vi "PurePursuit.vi"(0 "PathData":T2={"Path"=[{"x"=20.453371592539455, "y"=249.15925394548063}, {"x"=32.451138071473615, "y"=249.2417431099791}, {"x"=44.448056211953954, "y"=249.32366698389004}, {"x"=56.441768980000354, "y"=249.4040828136747}, {"x"=68.42823711154045, "y"=249.48106130123531}, {"x"=80.3987950137465, "y"=249.55036007485356}, {"x"=92.33398719870449, "y"=249.6026243647297}, {"x"=104.19073617112089, "y"=249.61714678939316}, {"x"=115.8737280283298, "y"=249.54805321076083}, {"x"=127.17183717836993, "y"=249.29372430937337}, {"x"=137.61733743281803, "y"=248.62905317811618}, {"x"=146.1740836060984, "y"=247.05537254809167}, {"x"=150.54675993154666, "y"=243.46800813008085}, {"x"=152.39728417160754, "y"=235.46668065740275}, {"x"=152.95934006523578, "y"=225.71717171741398}, {"x"=152.6076327980232, "y"=215.7198087862704}, {"x"=151.107691158904, "y"=206.8096834259849}, {"x"=147.4595538788043, "y"=201.04671193240875}, {"x"=139.23112896790275, "y"=198.5372634006921}, {"x"=128.93601727531555, "y"=197.49649482245655}, {"x"=117.71002861894719, "y"=197.11868334076806}, {"x"=106.06838831868264, "y"=197.04007755842468}, {"x"=94.24922045605804, "y"=197.09639645188625}, {"x"=82.37229762541514, "y"=197.21330877376334}, {"x"=70.51888885096747, "y"=197.35687893558043}, {"x"=58.78593931213765, "y"=197.51094316379152}, {"x"=47.350700340581184, "y"=197.66633376164685}, {"x"=36.58889694113597, "y"=197.8147673041893}, {"x"=27.32521119491603, "y"=197.9433223158581}, {"x"=21.38307030129124, "y"=198.025824964132}], "Spacing"=12.0}, 1 "SensorData":T3={"LeftDistance"=0.0, "RightDistance"=0.0, "LeftVelocity"=78.75762159095939, "RightVelocity"=-76.3848555077329, "Angle"=-0.01, "Location"={11.691968699047118, 248.03471515703785}}, 3 "Trackwidth":dbl=40.0 format="%#_13g", 5 "LookAhead":dbl=15.0, 7 "Reset":bool, 9 "MaxVel":dbl=40.0, 12 "Max Accel":dbl=50.0 format="%#_13g", 14 "Gains":T4={"FFV"=0.0088, "FFA"=0.0017, "Vel PID"={"P"=0.02, "I"=0.0, "D"=0.0}} {"Vel PID"."D" format="%.3f"; "Vel PID"."I" format="%.3f"; "Vel PID"."P" format="%.3f"}) -> (2 "Graph":cluster{cluster{"x":dbl, "y":dbl}[]}[](graph)=[{[{"x"=20.453371592539455, "y"=249.15925394548063}, {"x"=32.451138071473615, "y"=249.2417431099791}, {"x"=44.448056211953954, "y"=249.32366698389004}, {"x"=56.441768980000354, "y"=249.4040828136747}, {"x"=68.42823711154045, "y"=249.48106130123531}, {"x"=80.3987950137465, "y"=249.55036007485356}, {"x"=92.33398719870449, "y"=249.6026243647297}, {"x"=104.19073617112089, "y"=249.61714678939316}, {"x"=115.8737280283298, "y"=249.54805321076083}, {"x"=127.17183717836993, "y"=249.29372430937337}, {"x"=137.61733743281803, "y"=248.62905317811618}, {"x"=146.1740836060984, "y"=247.05537254809167}, {"x"=150.54675993154666, "y"=243.46800813008085}, {"x"=152.39728417160754, "y"=235.46668065740275}, {"x"=152.95934006523578, "y"=225.71717171741398}, {"x"=152.6076327980232, "y"=215.7198087862704}, {"x"=151.107691158904, "y"=206.8096834259849}, {"x"=147.4595538788043, "y"=201.04671193240875}, {"x"=139.23112896790275, "y"=198.5372634006921}, {"x"=128.93601727531555, "y"=197.49649482245655}, {"x"=117.71002861894719, "y"=197.11868334076806}, {"x"=106.06838831868264, "y"=197.04007755842468}, {"x"=94.24922045605804, "y"=197.09639645188625}, {"x"=82.37229762541514, "y"=197.21330877376334}, {"x"=70.51888885096747, "y"=197.35687893558043}, {"x"=58.78593931213765, "y"=197.51094316379152}, {"x"=47.350700340581184, "y"=197.66633376164685}, {"x"=36.58889694113597, "y"=197.8147673041893}, {"x"=27.32521119491603, "y"=197.9433223158581}, {"x"=21.38307030129124, "y"=198.025824964132}]}, {[{"x"=11.691968699047118, "y"=248.03471515703785}, {"x"=23.691968516276667, "y"=248.03680955212963}]}, {[{"x"=152.95934006523578, "y"=225.71717171741398}]}, {[{"x"=26.691968699047116, "y"=248.03471515703785}, {"x"=25.95781644347442, "y"=252.66997007266207}, {"x"=23.827223614671333, "y"=256.85149394142496}, {"x"=20.508747483434213, "y"=260.16997007266207}, {"x"=16.32722361467133, "y"=262.3005629014651}, {"x"=11.69196869904712, "y"=263.03471515703785}, {"x"=7.056713783422908, "y"=262.3005629014651}, {"x"=2.875189914660023, "y"=260.16997007266207}, {"x"=-0.4432862165770928, "y"=256.85149394142496}, {"x"=-2.5738790453801847, "y"=252.66997007266207}, {"x"=-3.308031300952882, "y"=248.03471515703785}, {"x"=-2.5738790453801865, "y"=243.39946024141364}, {"x"=-0.44328621657709455, "y"=239.21793637265077}, {"x"=2.8751899146600195, "y"=235.89946024141364}, {"x"=7.056713783422905, "y"=233.76886741261055}, {"x"=11.691968699047115, "y"=233.03471515703785}, {"x"=16.327223614671325, "y"=233.76886741261055}, {"x"=20.508747483434213, "y"=235.89946024141364}, {"x"=23.82722361467133, "y"=239.21793637265074}, {"x"=25.95781644347442, "y"=243.39946024141364}, {"x"=26.691968699047116, "y"=248.03471515703785}]}, {[{"x"=16.728162111415877, "y"=242.99940064954055}, {"x"=16.48171627411582, "y"=244.55539842807914}, {"x"=15.766502597859695, "y"=245.95908430278035}, {"x"=14.652531180466154, "y"=247.0730557201739}, {"x"=13.248845305764926, "y"=247.78826939643002}, {"x"=11.692847527226334, "y"=248.03471523373008}, {"x"=10.136849748687744, "y"=247.78826939643002}, {"x"=8.733163873986515, "y"=247.0730557201739}, {"x"=7.619192456592972, "y"=245.95908430278035}, {"x"=6.903978780336848, "y"=244.55539842807914}, {"x"=6.6575329430367916, "y"=242.99940064954055}, {"x"=6.903978780336848, "y"=241.44340287100195}, {"x"=7.619192456592971, "y"=240.03971699630074}, {"x"=8.733163873986513, "y"=238.9257455789072}, {"x"=10.136849748687743, "y"=238.21053190265107}, {"x"=11.692847527226332, "y"=237.964086065351}, {"x"=13.248845305764924, "y"=238.21053190265107}, {"x"=14.652531180466152, "y"=238.9257455789072}, {"x"=15.766502597859695, "y"=240.03971699630074}, {"x"=16.48171627411582, "y"=241.44340287100195}, {"x"=16.728162111415877, "y"=242.99940064954055}]}], 4 "LeftValue":dbl=2.7501251582780792, 6 "RightValue":dbl=-2.0461251582780795, 8 "TargetVel":dbl=40.0, 10 "Done":bool)   [LabVIEW 2017]
doc: "Takes in encoder and gyro data, and a path. In real time, calculates the left and right power to send to the motors to travel the path at a specified max speed, acceleration, and lookahead distance"
panel:
  in  "Speed/Curve":dbl=3.0 format="%#_13g"
  in  "Max dx/dt":dbl=10.0 format="%#_13g"
  out "TargetVelGraph":dbl(graph)
  out "Waveform Chart":T1(graph)={"l"=198.87785889523798, "dx/dt"=78.75762159095939, "r"=-118.87785889523798, "dx/dt"=-76.3848555077329}
  in  "Average Vels":bool
  # "SET DEFAULTS"
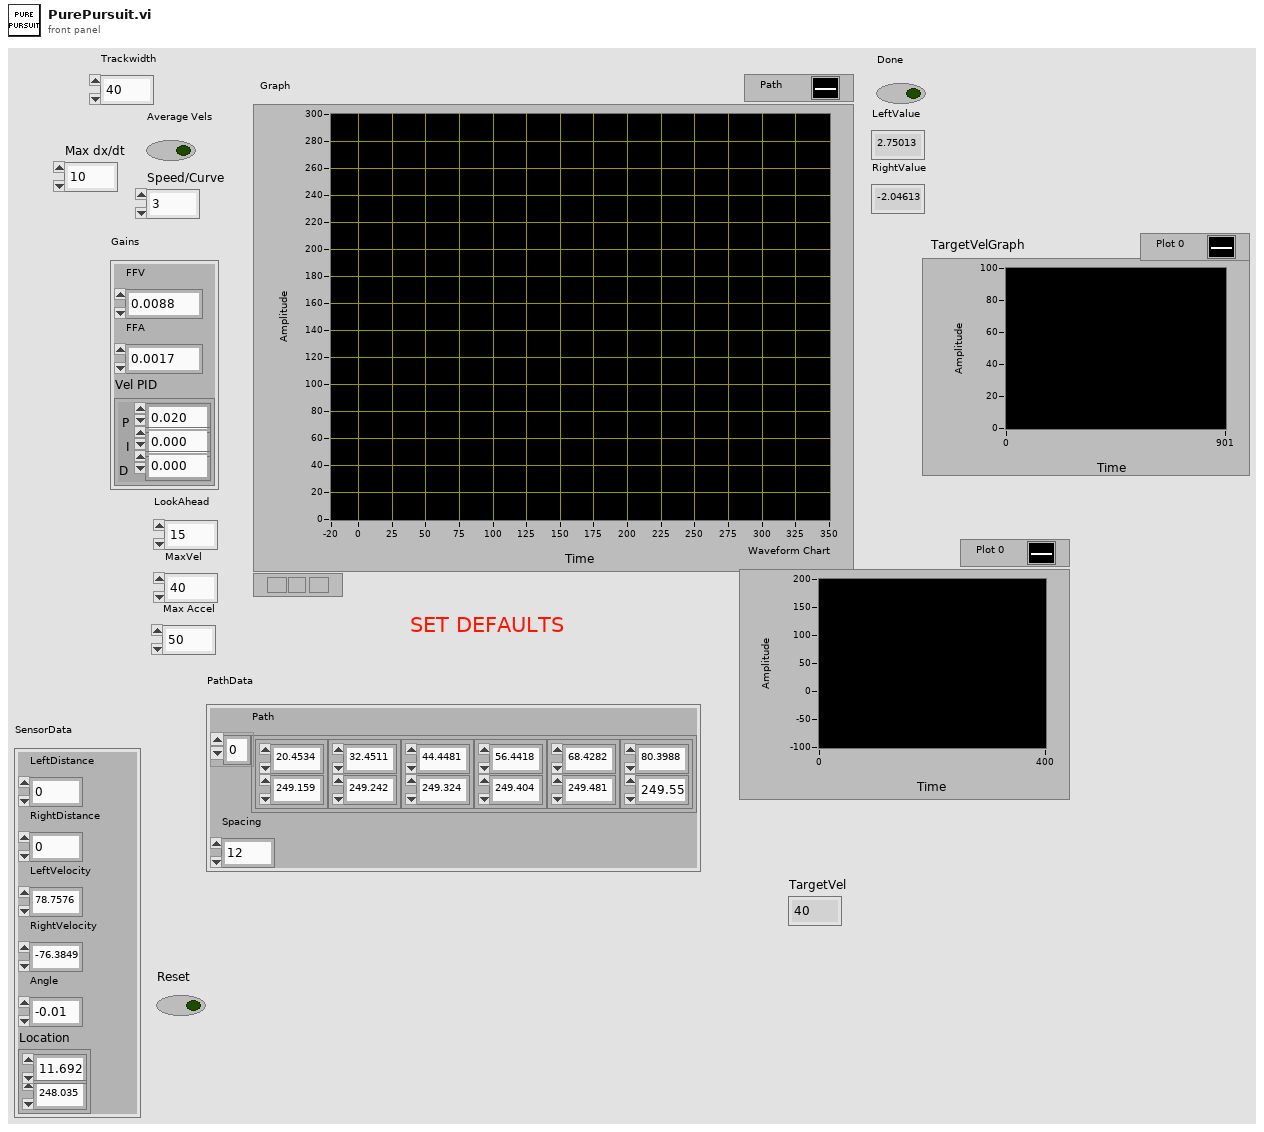
[diagram p1: front panel]
types:
  T1 = cluster{"l":dbl, "dx/dt":dbl, "r":dbl, "dx/dt":dbl}
  T2 = cluster{"Path":cluster{"x":dbl, "y":dbl}[], "Spacing":dbl}
  T3 = cluster{"LeftDistance":dbl, "RightDistance":dbl, "LeftVelocity":dbl, "RightVelocity":dbl, "Angle":dbl, "Location":cluster{dbl, dbl}}
  T4 = cluster{"FFV":dbl, "FFA":dbl, "Vel PID":cluster{"P":dbl, "I":dbl, "D":dbl}}
  T5 = cluster{"Path":cluster{"x":dbl, "y":dbl}[], "Spacing":dbl, "DistancesToEnd":dbl[], "Vel":dbl[]}
  T6 = cluster{"l":dbl, "LeftVelocity":dbl, "r":dbl, "RightVelocity":dbl}
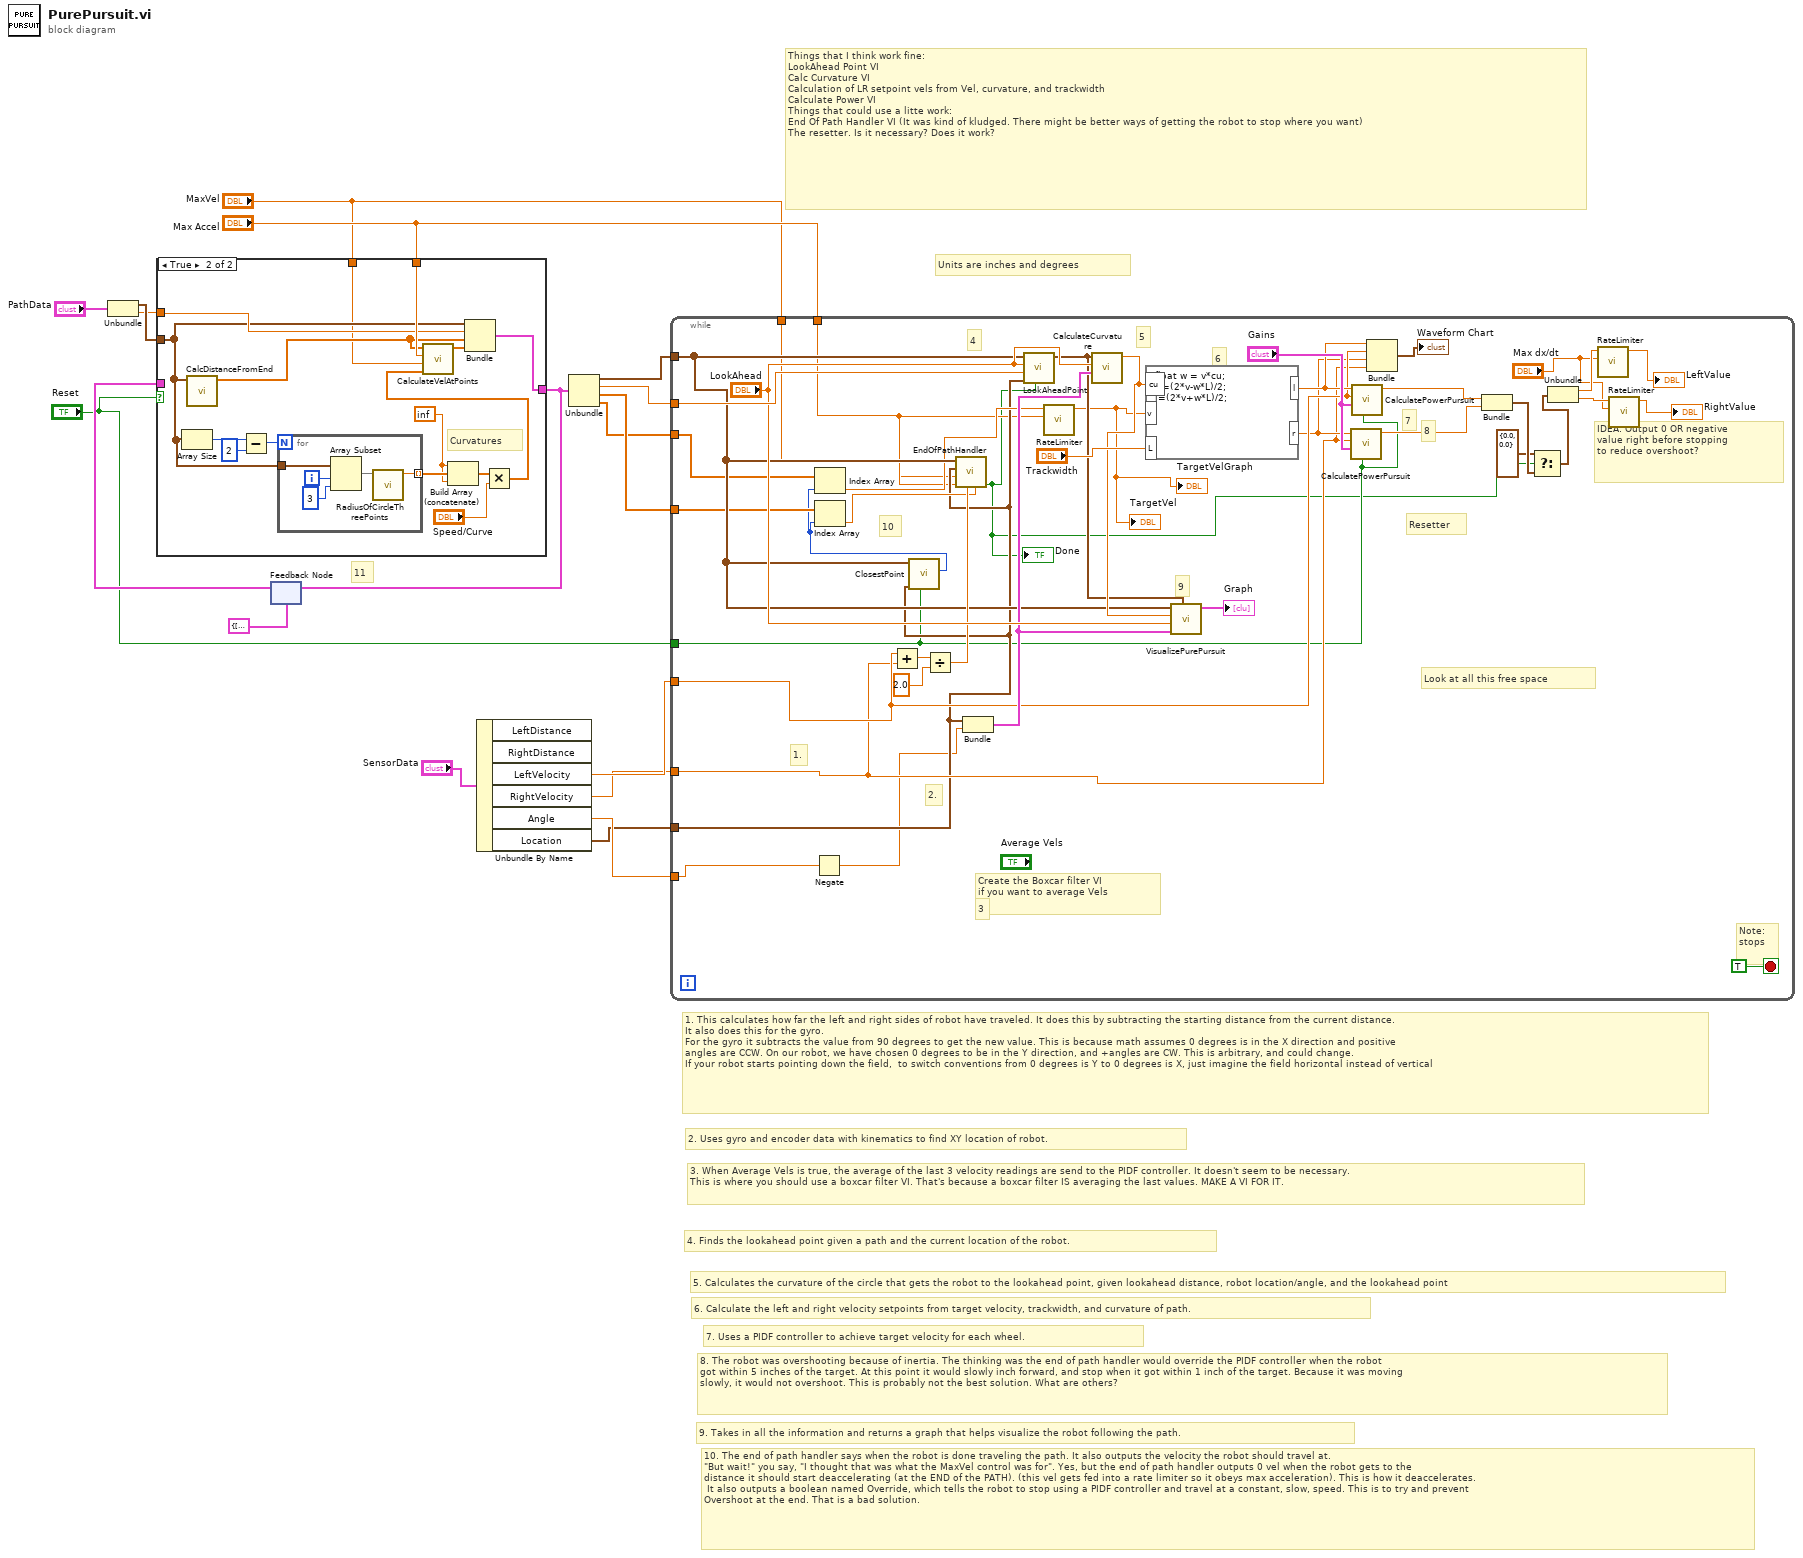
[diagram p0: block diagram]
diagram:
  # "11"
  # "10. The end of path handler says when the robot is done traveling the path. It also outputs the velocity the robot should travel at.\n\"But wait!\" you say, \"I thought that was what the MaxVel control was for\". Yes, but the end of path handler outputs 0 vel when the robot gets to the\ndistance it should start deaccelerating (at the END of the PATH). (this vel gets fed into a rate limiter so it obeys max acceleration). This is how it deaccelerates. \n It also outputs a boolean named Override, which tells the robot to stop using a PIDF controller and travel at a constant, slow, speed. This is to try and prevent\nOvershoot at the end. That is a bad solution."
  # "9. Takes in all the information and returns a graph that helps visualize the robot following the path."
  # "8. The robot was overshooting because of inertia. The thinking was the end of path handler would override the PIDF controller when the robot\ngot within 5 inches of the target. At this point it would slowly inch forward, and stop when it got within 1 inch of the target. Because it was moving\nslowly, it would not overshoot. This is probably not the best solution. What are others?"
  # "7. Uses a PIDF controller to achieve target velocity for each wheel."
  # "6. Calculate the left and right velocity setpoints from target velocity, trackwidth, and curvature of path."
  # "Things that I think work fine:\nLookAhead Point VI\nCalc Curvature VI\nCalculation of LR setpoint vels from Vel, curvature, and trackwidth\nCalculate Power VI\nThings that could use a litte work:\nEnd Of Path Handler VI (It was kind of kludged. There might be better ways of getting the robot to stop where you want)\nThe resetter. Is it necessary? Does it work?"
  # "Units are inches and degrees"
  # "5. Calculates the curvature of the circle that gets the robot to the lookahead point, given lookahead distance, robot location/angle, and the lookahead point"
  # "4. Finds the lookahead point given a path and the current location of the robot."
  # "3. When Average Vels is true, the average of the last 3 velocity readings are send to the PIDF controller. It doesn't seem to be necessary.\nThis is where you should use a boxcar filter VI. That's because a boxcar filter IS averaging the last values. MAKE A VI FOR IT."
  # "2. Uses gyro and encoder data with kinematics to find XY location of robot."
  # "1. This calculates how far the left and right sides of robot have traveled. It does this by subtracting the starting distance from the current distance.\nIt also does this for the gyro.\nFor the gyro it subtracts the value from 90 degrees to get the new value. This is because math assumes 0 degrees is in the X direction and positive\nangles are CCW. On our robot, we have chosen 0 degrees to be in the Y direction, and +angles are CW. This is arbitrary, and could change.\nIf your robot starts pointing down the field,  to switch conventions from 0 degrees is Y to 0 degrees is X, just imagine the field horizontal instead of vertical"
  n1 = Unbundle("PathData") -> ("Path"=w3:cluster{"x":dbl, "y":dbl}[], "Spacing"=w2:dbl)
  n2 = feedback #1(T5 {"Path"=[{"x"=0.0, "y"=0.0}, {"x"=0.0, "y"=46.0}, {"x"=77.25, "y"=97.5}], "Spacing"=0.0, "DistancesToEnd"=[309.52253206522465, 306.5225388483889, 303.52254576348514, 300.5225494135135, 297.5225482930251, 294.5225431892043, 291.52253649479525, 288.5225309404311, 285.52252839669825, 282.52252922985826, 279.52253236801363, 276.5225359199274, 273.5225380077533, 270.5225374640896, 267.5225341651582, 264.5225289486152, 261.52252321975885, 258.52251843460203, 255.52251565052453, 252.52251527415513, 249.52251704698162, 246.52252022727612, 243.52252387624657, 240.5225271449837, 237.52252948071848, 234.5225307115883, 231.5225310121264, 228.5225307841412, 225.52253050297352, 222.52253057724883, 219.522531255923, 216.52253259658312, 213.5225344902357, 210.52253672481638, 207.52253906428678, 204.52254132188853, 201.52254341264756, 198.5225453787386, 195.52254738922483, 192.52254972128023, 189.5225527326013, 186.5225568345679, 183.5225624736694, 180.52257012582595, 177.52258030545136, 174.52259358906986, 171.52261065227918, 168.52263231879937, 165.52265962102405, 162.52269387257934, 159.52273675466557, 156.52279041923995, 153.52285761342083, 150.52294183093122, 147.52304749810799, 144.52318020416902, 141.5233469881785, 138.52355669860665, 135.52382044572104, 132.52415217017628, 129.52456938475245, 126.52509392552396, 123.52575388229783, 120.52658224756205, 117.52762599636499, 114.52893466674816, 111.5305811433295, 108.53265099247815, 105.5352499693053, 102.53851522329074, 99.54261858949184, 96.54777258499563, 93.55424339621041, 90.56236601643654, 87.57255952674781, 84.58534501572932, 81.60137180227034, 78.62143961905741, 75.64655567097594, 72.6779255489502, 69.71706974165639, 66.76578984976493, 63.82625595622302, 60.90103565379168, 57.99306437227732, 55.10557379235981, 52.24189700353533, 49.40502603383819, 46.59675379579783, 43.81612021857386, 41.056705992040605, 38.30212773163372, 35.53590323835957, 32.752089130751756, 29.950811925036337, 27.135602619179224, 24.311917874683846, 21.486403150766286, 18.666614193530503, 15.861028930660632, 13.07925664424869, 10.33239795871144, 7.633538890247935, 4.998382632368401, 2.4460384085185156, 0.0], "Vel"=[309.52253206522465, 306.5225388483889, 303.52254576348514, 300.5225494135135, 297.5225482930251, 294.5225431892043, 291.52253649479525, 288.5225309404311, 285.52252839669825, 282.52252922985826, 279.52253236801363, 276.5225359199274, 273.5225380077533, 270.5225374640896, 267.5225341651582, 264.5225289486152, 261.52252321975885, 258.52251843460203, 255.52251565052453, 252.52251527415513, 249.52251704698162, 246.52252022727612, 243.52252387624657, 240.5225271449837, 237.52252948071848, 234.5225307115883, 231.5225310121264, 228.5225307841412, 225.52253050297352, 222.52253057724883, 219.522531255923, 216.52253259658312, 213.5225344902357, 210.52253672481638, 207.52253906428678, 204.52254132188853, 201.52254341264756, 198.5225453787386, 195.52254738922483, 192.52254972128023, 189.5225527326013, 186.5225568345679, 183.5225624736694, 180.52257012582595, 177.52258030545136, 174.52259358906986, 171.52261065227918, 168.52263231879937, 165.52265962102405, 162.52269387257934, 159.52273675466557, 156.52279041923995, 153.52285761342083, 150.52294183093122, 147.52304749810799, 144.52318020416902, 141.5233469881785, 138.52355669860665, 135.52382044572104, 132.52415217017628, 129.52456938475245, 126.52509392552396, 123.52575388229783, 120.52658224756205, 117.52762599636499, 114.52893466674816, 111.5305811433295, 108.53265099247815, 105.5352499693053, 102.53851522329074, 99.54261858949184, 96.54777258499563, 93.55424339621041, 90.56236601643654, 87.57255952674781, 84.58534501572932, 81.60137180227034, 78.62143961905741, 75.64655567097594, 72.6779255489502, 69.71706974165639, 66.76578984976493, 63.82625595622302, 60.90103565379168, 57.99306437227732, 55.10557379235981, 52.24189700353533, 49.40502603383819, 46.59675379579783, 43.81612021857386, 41.056705992040605, 38.30212773163372, 35.53590323835957, 32.752089130751756, 29.950811925036337, 27.135602619179224, 24.311917874683846, 21.486403150766286, 18.666614193530503, 15.861028930660632, 13.07925664424869, 10.33239795871144, 7.633538890247935, 4.998382632368401, 2.4460384085185156, 0.0]} ("PathData")) -> (w8:T5)
  n3 = case shown="True" "Reset" {
    tunnel: [w19 w31] -> w7
    tunnel: w8 -> [w19 _]
    tunnel: "Max Accel" -> [_ w33]
    tunnel: "MaxVel" -> [_ w21]
    tunnel: w3 -> [_ w23]
    tunnel: w2 -> [_ w32]
    frame False {
    }
    frame True {
      w25 = inf
      # "Curvatures"
      n4 = Array Size(array=w23) -> (size(s)=w27:i32)
      n5 = call "CalcDistanceFromEnd.vi"("Path"=w23) -> ("DistancesToEnd"=w22:dbl[])  [unwired: 10 in]
      n6 = Subtract(x=w27, y=2) -> (x-y=w28:i32)
      n7 = for {
        N: w28 -> [_]
        tunnel: w23 -> [w39]
        tunnel: [w35] -> w29 mode=indexing
        i -> [w38]
        n8 = Array Subset(array=w39, index=w38, length=3) -> (w36:cluster{"x":dbl, "y":dbl}[])
        n9 = call "RadiusOfCircleThreePoints.vi"("Points"=w36) -> ("R"=w35:dbl)  [unwired: 10 in]
      }
      n10 = Build Array (concatenate)(w25, w29, w25) -> (w30:dbl[])
      n11 = Multiply(x=w30, y="Speed/Curve") -> (x*y=w20:dbl[])
      n12 = call "CalculateVelAtPoints.vi"("MaxVels"=w20, "MaxVel"=w21, "MaxAccel"=w33, "DistancesToEnd"=w22) -> ("Vel"=w34:dbl[])  [unwired: 7 in]
      n13 = Bundle("Path"=w23, "Spacing"=w32, "DistancesToEnd"=w22, "Vel"=w34) -> (w31:T5)  [unwired: 1 in]
    }
  }
  n14 = feedback-in #1(w7) -> ()
  n15 = Unbundle By Name("SensorData") -> ("LeftVelocity"=w17:dbl, "RightVelocity"=w16:dbl, "Angle"=w11:dbl, "Location"=w10:cluster{dbl, dbl})  [unwired: 2 out]
  n16 = Unbundle(w7) -> ("Path"=w15:cluster{"x":dbl, "y":dbl}[], "Spacing"=w14:dbl, "DistancesToEnd"=w13:dbl[], "Vel"=w12:dbl[])
  n17 = while {
    tunnel: w15 -> [w62]
    tunnel: w14 -> [w80]
    tunnel: w17 -> [w65]
    tunnel: w16 -> [w63]
    tunnel: w11 -> [w49]
    tunnel: w13 -> [w60]
    tunnel: w12 -> [w58]
    tunnel: w10 -> [w52]
    tunnel: "Max Accel" -> [w51]
    tunnel: "MaxVel" -> [w50]
    tunnel: "Reset" -> [w47]
    stop <- TRUE stop-if-true
    # "Create the Boxcar filter VI\nif you want to average Vels"
    # "Look at all this free space"
    # "Note:\nstops"
    # "IDEA: Output 0 OR negative\nvalue right before stopping\nto reduce overshoot?"
    # "10"
    # "9"
    # "8"
    # "7"
    # "6"
    # "5"
    # "4"
    # "3"
    # "2."
    # "1."
    # "Resetter"
    n18 = Negate(x=w49) -> (-x=w48:dbl)
    n19 = Add(x=w65, y=w63) -> (x+y=w71:dbl)
    n20 = call "ClosestPoint.vi"("Reset"=w47, "Robot"=w52, "Path"=w62) -> ("ClosestIndex"=w57:i32)  [unwired: 7 in, 1 out]
    n21 = Index Array(array=w58, index=w57) -> (element=w56:dbl)
    n22 = Index Array(array=w60, index=w57) -> (element=w59:dbl)
    n23 = Divide(x=w71, y=2.0) -> (x/y=w69:dbl)
    n24 = call "EndOfPathHandler.vi"("DistanceToEnd"=w59, "CurrentVel"=w69, "MaxAccel"=w51, "MaxVel"=w50, "RobotLocation"=w52, "Path"=w62) -> ("Done"=w46:bool)  [unwired: 2 in, 3 out]
    "Done" <- w46
    n25 = Bundle("Location"=w52, w48) -> (w75:cluster{"Location":cluster{dbl, dbl}, dbl})  [unwired: 1 in]
    n26 = call "LookAheadPoint.vi"("Reset"=w46, "Robot"=w52, "Spacing"=w80, "LookAhead"="LookAhead", "Path"=w62) -> ("Point"=w74:cluster{"x":dbl, "y":dbl})  [unwired: 5 in, 1 out]
    n27 = call "RateLimiter.vi"("Max dx/dt"=w51, "Input"=w56) -> ("Output"=w45:dbl)  [unwired: 9 in]
    "TargetVel" <- w45
    "TargetVelGraph" <- w45
    n28 = call "CalculateCurvature.vi"("Robot"=w75, "Lookahead"="LookAhead", "Point"=w74) -> ("Curvature"=w77:dbl)  [unwired: 8 in]
    n29 = formula code="float w = v*cu;\nr =(2*v-w*L)/2;\nl=(2*v+w*L)/2;"("L"="Trackwidth", "cu"=w77, "v"=w45) -> ("r"=w64:dbl, "l"=w67:dbl)
    n30 = call "VisualizePurePursuit.vi"("Lookahead Point"=w74, "Robot"=w75, "Lookahead"="LookAhead", "Curvature"=w77, "Path"=w62) -> ("Graph"=→"Graph":cluster{cluster{"x":dbl, "y":dbl}[]}[])  [unwired: 6 in]
    n31 = call "CalculatePowerPursuit.vi"("Reset"=w47, "Gains"="Gains", "Vel"=w63, "Target Vel"=w64) -> ("Power"=w72:dbl)  [unwired: 7 in]
    n32 = call "CalculatePowerPursuit.vi"("Reset"=w47, "Gains"="Gains", "Vel"=w65, "Target Vel"=w67) -> ("Power"=w73:dbl)  [unwired: 7 in]
    n33 = Bundle("l"=w67, "LeftVelocity"=w65, "r"=w64, "RightVelocity"=w63) -> (→"Waveform Chart":T6)  [unwired: 1 in]
    n34 = Bundle("Power"=w73, "Power"=w72) -> (w55:cluster{"Power":dbl, "Power":dbl})  [unwired: 1 in]
    n35 = Select(t=cluster{"Power":dbl, "Power":dbl} {"Power"=0.0, "Power"=0.0}, s=w46, f=w55) -> (s? t:f=w53:cluster{"Power":dbl, "Power":dbl})
    n36 = Unbundle(w53) -> ("Power"=w44:dbl, "Power"=w43:dbl)
    n37 = call "RateLimiter.vi"("Max dx/dt"="Max dx/dt", "Input"=w44) -> ("Output"=→"LeftValue":dbl)  [unwired: 9 in]
    n38 = call "RateLimiter.vi"("Max dx/dt"="Max dx/dt", "Input"=w43) -> ("Output"=→"RightValue":dbl)  [unwired: 9 in]
  }
